vi "Set_API_Description.vi"(1 "Description":string, 2 "Argument List In":string[](array[string])) -> (0 "Argument List Out":string[](array[string]))   [LabVIEW 2011]
doc: "This VI sets an API descriptor via the \"Argument List\" parameters. The API description will be displayed in parantheses next to the corresponding event in the Growth Sequence Editor."
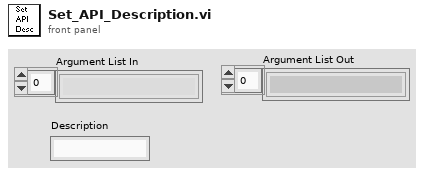
[diagram p1: front panel]
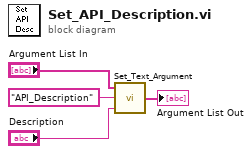
[diagram p0: block diagram]
diagram:
  n1 = call "Set_Text_Argument.vi"("Text"="Description", "Argument"="API_Description", "Argument List In"="Argument List In") -> ("Argument List Out"=→"Argument List Out":string[])
